vi "specu1a 1.0.0 Read User EEPROM.vi"(0 "Device Handle":i32, 1 "Address":u16, 3 "error in (no error)":errorcluster, 4 "Length":u16=256) -> (5 "Device Handle out":i32, 6 "EEPROM String":string, 7 "error out":errorcluster)   [LabVIEW 2010]
uses:
  WINDOWS/SYSTEM32/DRIVERS/specu1a.dll
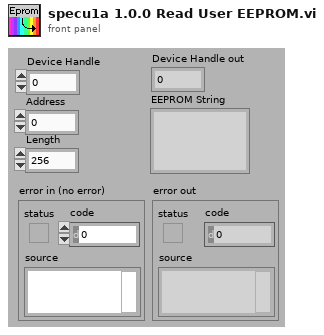
[diagram p1: front panel]
types:
  T1 = cluster{"[0]":u8, "[1]":u8, "[2]":u8, "[3]":u8, "[4]":u8, "[5]":u8, "[6]":u8, "[7]":u8, "[8]":u8, "[9]":u8, "[10]":u8, "[11]":u8, "[12]":u8, "[13]":u8, "[14]":u8, "[15]":u8, "[16]":u8, "[17]":u8, "[18]":u8, "[19]":u8, "[20]":u8, "[21]":u8, "[22]":u8, "[23]":u8, "[24]":u8, "[25]":u8, "[26]":u8, "[27]":u8, "[28]":u8, "[29]":u8, "[30]":u8, "[31]":u8, "[32]":u8, "[33]":u8, "[34]":u8, "[35]":u8, "[36]":u8, "[37]":u8, "[38]":u8, "[39]":u8, "[40]":u8, "[41]":u8, "[42]":u8, "[43]":u8, "[44]":u8, "[45]":u8, "[46]":u8, "[47]":u8, "[48]":u8, "[49]":u8, "[50]":u8, "[51]":u8, "[52]":u8, "[53]":u8, "[54]":u8, "[55]":u8, "[56]":u8, "[57]":u8, "[58]":u8, "[59]":u8, "[60]":u8, "[61]":u8, "[62]":u8, "[63]":u8}
  T2 = typedef "specu1a 1.0.0 Error codes.ctl" = enum16{"INVALID_HANDLE_VALUE", "USBDEV_SUCCESS", "USBDEV_INVALID_HANDLE", "USBDEV_UNSUCCESS", "USBDEV_INVALID_VALUE", "USBDEV_CHECK_NORMAL", "USBDEV_CHECK_INVALID", "USBDEV_CHECK_REMOVE", "USBDEV_CHECK_OTHER", "USBDEV_RESET_ERROR", "USBDEV_BULKSIZE_ERROR", "USBDEV_BULK_READ_ERROR", "USBDEV_BULK_NOT_UPDATED", "USBDEV_TIME_OVER_ERROR", "USBDEV_TIME_UNDER_ERROR", "USBDEV_TIME_SET_ERROR", "USBDEV_SET_GAIN_ERROR", "USBDEV_GET_TEMP_ERROR", "USBDEV_SET_TRIGGER_ERROR", "USBDEV_RW_EEP_ADDR_ERROR", "USBDEV_RW_EEP_SIZE_ERROR", "USBDEV_RW_EEP_OVER_ERROR", "USBDEV_RW_EEP_ERROR", "UNITID_PRODUCTID_CONFLICT", "UNKNOWN_ERROR"}
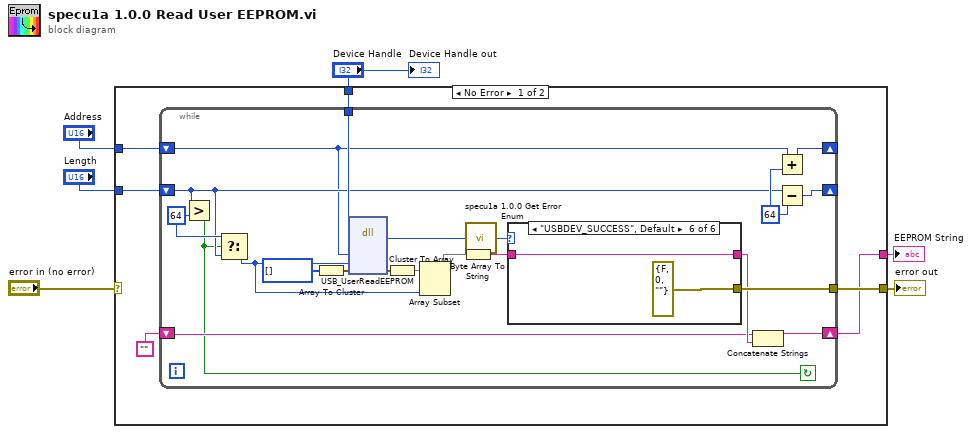
[diagram p0: block diagram]
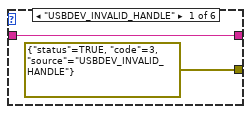
[diagram p2: hidden frame]
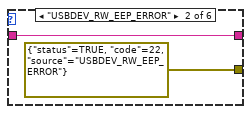
[diagram p3: hidden frame]
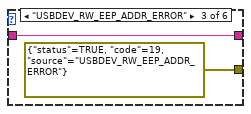
[diagram p4: hidden frame]
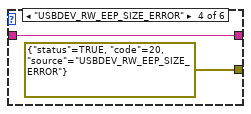
[diagram p5: hidden frame]
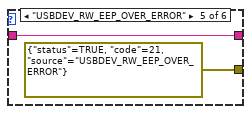
[diagram p6: hidden frame]
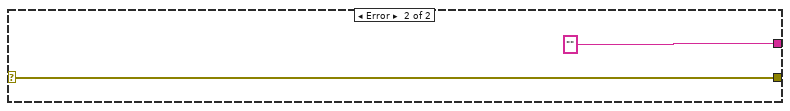
[diagram p7: hidden frame]
diagram:
  n1 = case shown="No Error" "error in (no error)" {
    selector: "error in (no error)" -> [_ w47]
    tunnel: [w12 w47] -> w5
    tunnel: "Device Handle" -> [w11 _]
    tunnel: "Length" -> [w10 _]
    tunnel: [w8 "" ("string")] -> w2
    tunnel: "Address" -> [w7 _]
    frame No Error {
      n2 = while {
        tunnel: [w33] -> w12
        tunnel: w11 -> [w32]
        shift-right: [w23] -> _
        shift-left: w10 -> [w17]
        shift-right: [w19] -> w8
        shift-left: "" -> [w18]
        shift-right: [w14] -> _
        shift-left: w7 -> [w13]
        stop <- w15 continue-if-true
        w21 = 64
        w22 = 64
        n3 = Greater?(x=w17, y=w22) -> (0:w15:bool)
        n4 = Select(t=w22, s=w15, f=w17) -> (s? t:f=w16:i32)
        n5 = Array To Cluster(array=u8[] []) -> (cluster=w29:T1)
        n6 = dll-call lib="C:/WINDOWS/SYSTEM32/DRIVERS/specu1a.dll" fn="USB_UserReadEEPROM" label="1.0.0 Read User EEPROM"("Device Handle"=w32, "Address"=w13, "Length"=w16, w29) -> (w28:u16, w27:T1)  [unwired: 6 in, 2 out]
        n7 = Cluster To Array(cluster=w27) -> (array=w26:u8[])
        n8 = Array Subset(array=w26, length=w16) -> (w25:u8[])  [unwired: 1 in]
        n9 = Byte Array To String(unsigned byte array=w25) -> (string=w24:string)
        n10 = call "specu1a 1.0.0 Get Error Enum.vi"("Error Code in"=w28) -> ("Specu1a 1.0.0 Error code out"=w31:T2)  [unwired: 4 in]
        n11 = case shown="\"USBDEV_SUCCESS\", Default" w31 {
          tunnel: [w34 w36 w38 w40 w42 w44] -> w20
          tunnel: [errorcluster {"status"=TRUE, "code"=3, "source"="USBDEV_INVALID_HANDLE"} ("error out") errorcluster {"status"=TRUE, "code"=22, "source"="USBDEV_RW_EEP_ERROR"} ("error out") errorcluster {"status"=TRUE, "code"=19, "source"="USBDEV_RW_EEP_ADDR_ERROR"} ("error out") errorcluster {"status"=TRUE, "code"=20, "source"="USBDEV_RW_EEP_SIZE_ERROR"} ("error out") errorcluster {"status"=TRUE, "code"=21, "source"="USBDEV_RW_EEP_OVER_ERROR"} ("error out") errorcluster {"status"=FALSE, "code"=0, "source"=""} ("error out")] -> w33
          tunnel: w24 -> [w34 w36 w38 w40 w42 w44]
          frame "USBDEV_INVALID_HANDLE" {
          }
          frame "USBDEV_RW_EEP_ERROR" {
          }
          frame "USBDEV_RW_EEP_ADDR_ERROR" {
          }
          frame "USBDEV_RW_EEP_SIZE_ERROR" {
          }
          frame "USBDEV_RW_EEP_OVER_ERROR" {
          }
          frame "USBDEV_SUCCESS", Default {
          }
        }
        n12 = Concatenate Strings(w18, w20) -> (w19:string)
        n13 = Add(x=w13, y=w21) -> (x+y=w14:i32)
        n14 = Subtract(x=w17, y=w21) -> (x-y=w23:i32)
      }
    }
    frame Error {
    }
  }
  "error out" <- w5
  "EEPROM String" <- w2
  "Device Handle out" <- "Device Handle"
